vi "PCAN_STATUS.vi"(7 "pathCAN_DLL":path, 8 "error in (no error)":errorcluster) -> (0 "error out":errorcluster, 3 "error":T1 items=["CAN_ERR_OK"=0, "CAN_ERR_XMTFULL"=1, "CAN_ERR_OVERRUN"=2, "CAN_ERR_BUSLIGHT"=4, "CAN_ERR_BUSHEAVY"=8, "CAN_ERR_BUSOFF"=16, "CAN_ERR_QRCVEMPTY"=32, "CAN_ERR_QOVERRUN"=64, "CAN_ERR_QXMTFULL"=128, "CAN_ERR_REGTEST"=256, "CAN_ERR_NOVXD"=512, "CAN_ERR_HWINUSE"=1024, "CAN_ERR_NETINUSE"=2048, "CAN_ERR_ILLHW"=5120, "CAN_ERR_ILLNET"=6144, "CAN_ERR_ILLCLINET"=7168, "CAN_ERR_RESOURCE"=8192, "CAN_ERR_ILLPARAMTYPE"=16384, "CAN_ERR_ILLPARAMVAL"=32768, "CAN_ERR_UNKNOWN"=65536])   [LabVIEW 2023, in "pCANLib.lvlib"]
uses:
  pCANLib.lvlib
  PCAN_ERROR.ctl
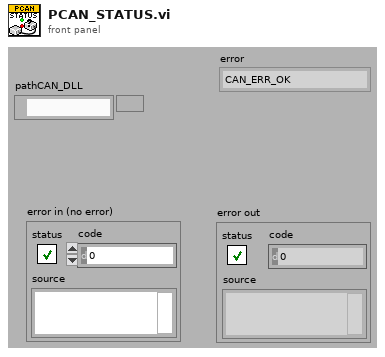
[diagram p1: front panel]
types:
  T1 = typedef "pCANLib.lvlib/PCAN_ERROR.ctl" = i32
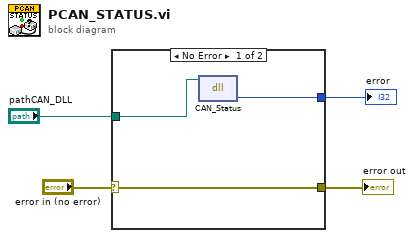
[diagram p0: block diagram]
diagram:
  n1 = case shown="No Error" "error in (no error)" {
    selector: "error in (no error)" -> [w6 w8]
    tunnel: [w7 _] -> w2
    tunnel: [w6 w8] -> w3
    tunnel: "pathCAN_DLL" -> [w5 _]
    frame No Error {
      n2 = dll-call lib="D:/PCAN/PCAN/PCAN Driver/PCAN_Driver/PCAN_USB.DLL" fn="CAN_Status"(path in=w5) -> ("return type"=w7:i32)  [unwired: 2 in, 2 out]
    }
    frame Error {
    }
  }
  "error out" <- w3
  "error" <- w2
